vi "getHologram.vi"(6 "Display":i32, 7 "session in":refnum<k35>, 8 "previous path":path, 9 "options cluster":T2, 10 "Beam in":T1, 11 "Hologram in":T1) -> (0 "error out":errorcluster, 1 "appended path":path, 2 "Beam out":T1, 3 "Hologram out":T1, 4 "file or folder exists?":bool)   [LabVIEW 2022 SP3]
uses:
  <vilib>/vision/Image Controls.llb/IMAQ Image.ctl
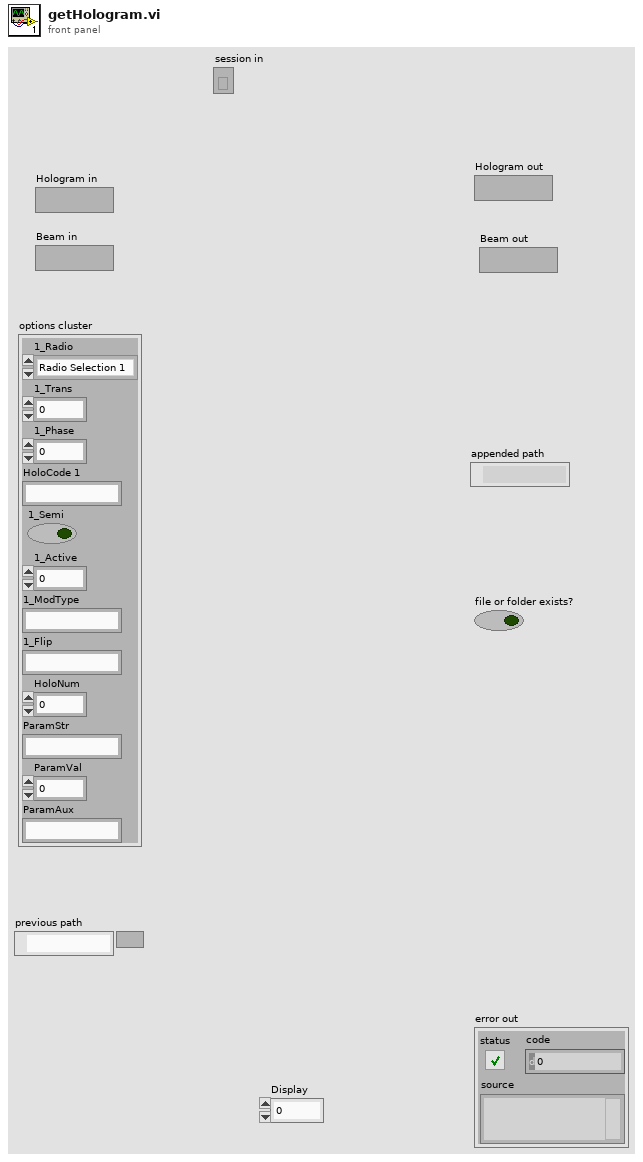
[diagram p1: front panel]
types:
  T1 = typedef "IMAQ Image.ctl" = refnum<image>
  T2 = cluster{"1_Radio":enum32{"Radio Selection 1", "Radio Selection 2", "Radio Selection 3", "Radio Selection 4", "Radio Selection 5", "Radio Selection 6", "Radio Selection 7", "Radio Selection 8"}, "1_Trans":dbl, "1_Phase":dbl, "HoloCode 1":string, "1_Semi":bool, "1_Active":u16, "1_ModType":string, "1_Flip":string, "HoloNum":dbl, "ParamStr":string, "ParamVal":dbl, "ParamAux":string}
  T3 = enum32{"Radio Selection 1", "Radio Selection 2", "Radio Selection 3", "Radio Selection 4", "Radio Selection 5", "Radio Selection 6", "Radio Selection 7", "Radio Selection 8"}
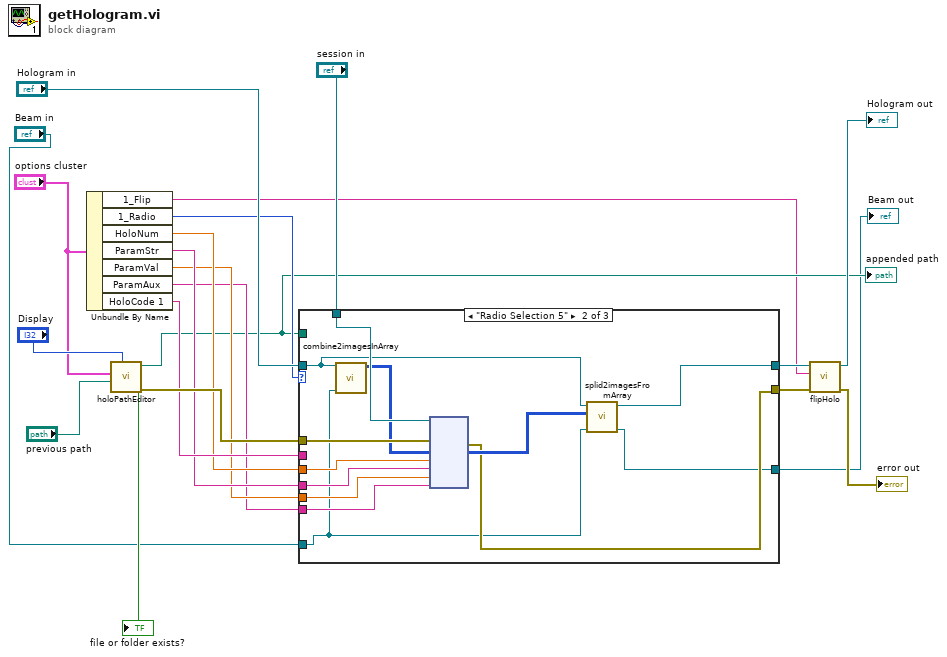
[diagram p0: block diagram]
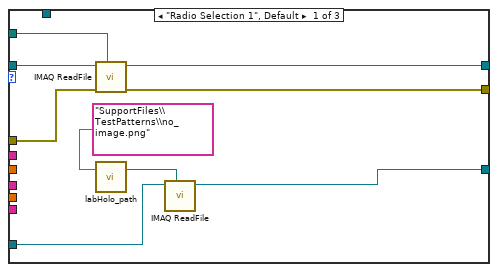
[diagram p2: hidden frame]
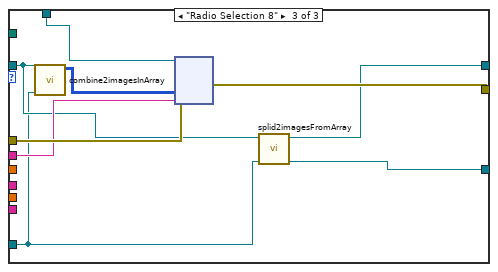
[diagram p3: hidden frame]
diagram:
  n1 = Unbundle By Name("options cluster") -> ("1_Flip"=w3:string, "1_Radio"=w10:T3, "HoloNum"=w8:dbl, "ParamStr"=w7:string, "ParamVal"=w6:dbl, "ParamAux"=w5:string, "HoloCode 1"=w9:string)
  n2 = call "holoPathEditor.vi"("Display"="Display", "prev. Path"="previous path", "input cluster"="options cluster") -> ("error out"=w14:errorcluster, "file or folder exists?"=→"file or folder exists?":bool, "appended path"=w4:path)  [unwired: 5 in, 1 out]
  "appended path" <- w4
  n3 = case shown="\"Radio Selection 5\"" w10 {
    tunnel: w4 -> [w30 _ _]
    tunnel: [w29 w34 w51] -> w17
    tunnel: [w26 w41 w48] -> w16
    tunnel: w14 -> [w28 w43 w52]
    tunnel: "Hologram in" -> [w27 w33 w46]
    tunnel: "session in" -> [_ w42 w50]
    tunnel: w9 -> [_ _ w49]
    tunnel: w8 -> [_ w40 _]
    tunnel: w7 -> [_ w39 _]
    tunnel: w6 -> [_ w38 _]
    tunnel: w5 -> [_ w37 _]
    tunnel: [w24 w32 w47] -> w2
    tunnel: "Beam in" -> [w25 w31 w44]
    frame "Radio Selection 1", Default {
      n4 = call "IMAQ ReadFile"("File Path"=w30, "error in (no error)"=w28, "Image"=w27) -> ("error out"=w29:errorcluster, "Image Out"=w26:T1)  [unwired: 4 in, 3 out]
      n5 = call "labHolo_path.vi"("sub folder or file (str)"="SupportFiles\\TestPatterns\\no_image.png") -> ("labHolo path"=w22:path)  [unwired: 1 in, 1 out]
      n6 = call "IMAQ ReadFile"("File Path"=w22, "Image"=w25) -> ("Image Out"=w24:T1)  [unwired: 5 in, 4 out]
    }
    frame "Radio Selection 5" {
      n7 = call "combine2imagesInArray.vi"("Beam in"=w31, "Image in"=w33) -> ("Array"=w36:u8[][][])  [unwired: 9 in]
      n8 = node(w42, w43, w36, w40, w39, w38, w37) -> (w34:errorcluster, w35:u8[][][])  [unwired: 6 in, 3 out]
      n9 = call "splid2imagesFromArray.vi"("Beam in"=w31, "Combined array"=w35, "Image in"=w33) -> ("Beam Out"=w32:T1, "Image out"=w41:T1)  [unwired: 7 in]
    }
    frame "Radio Selection 8" {
      n10 = call "combine2imagesInArray.vi"("Beam in"=w44, "Image in"=w46) -> ("Array"=w45:u8[][][])  [unwired: 9 in]
      n11 = node(w50, w52, w45, w49) -> (w51:errorcluster)  [unwired: 4 in, 3 out]
      n12 = call "splid2imagesFromArray.vi"("Beam in"=w44, "Image in"=w46) -> ("Beam Out"=w47:T1, "Image out"=w48:T1)  [unwired: 8 in]
    }
  }
  "Beam out" <- w2
  n13 = call "flipHolo.vi"("error in (no error)"=w17, "flip_option"=w3, "Image in"=w16) -> ("error out"=→"error out":errorcluster, "Image out"=→"Hologram out":T1)  [unwired: 7 in]
